vi "SyncParameters.vi"(4 "Excitation":T1={"Frequency"=1000.0, "Amplitude"=5e-07, "DC Offset"=0.0, "Cut Off"=40.0, "RaPF"=FALSE, "Shift"=0.0} {"Shift" min=-100.0 max=100.0 format="%_1p%"}, 6 "lineFitThreshold":dbl, 7 "inputSensitivity":dbl, 8 "error in":errorcluster, 9 "syncParameters":T4, 10 "BackgroundParameters":T3, 11 "FPGA VI Reference In":T2) -> (0 "error out":errorcluster, 3 "FPGA VI Reference Out":T2)   [LabVIEW 2016]
uses:
  controls/FPGAVIreferenceTypeDef.ctl
  controls/Enum.ctl
  <vilib>/Utility/error.llb/Error Cluster From Error Code.vi
  <vilib>/rvi/errors/niLvFpgaAdjustHostInterfaceError.vi
  <vilib>/rvi/interface/nirviReadWriteControl/nirviReadWriteControl.xnode
  FPGA Bitfiles/qnmController797_usbRIO_controllerFPGAmu.lvbitx
  NiFpgaLv.dll
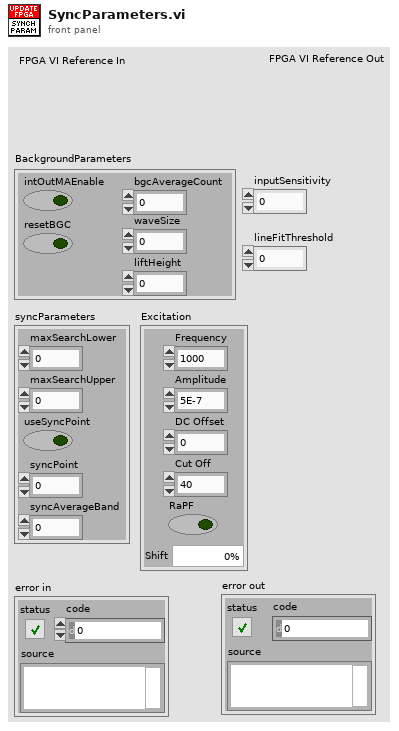
[diagram p1: front panel]
types:
  T1 = cluster{"Frequency":dbl, "Amplitude":dbl, "DC Offset":dbl, "Cut Off":dbl, "RaPF":bool, "Shift":dbl}
  T2 = typedef "FPGAVIreferenceTypeDef.ctl" = refnum<k20>
  T3 = cluster{"intOutMAEnable":bool, "bgcAverageCount":u16, "waveSize":u32, "resetBGC":bool, "liftHeight":fxp<+/-,15,4>}
  T4 = cluster{"maxSearchLower":u16, "maxSearchUpper":u16, "useSyncPoint":bool, "syncPoint":u16, "syncAverageBand":u16}
  T5 = typedef "Enum.ctl" = enum16{"Init", "Read", "Write"}
  T6 = cluster{"maxSearchLower":u16, "maxSearchUpper":u16}
  T7 = cluster{"ort.p.winSizeP2":u16, "ort.p.syncPoint":u16, "ort.p.useSyncPoint":bool, "ort.p.bypassAvg":bool, "ort.p.searchBounds":cluster{"maxSearchLower":u16, "maxSearchUpper":u16}}
  T8 = cluster{"maxLoc":u16, "threshold":i16, "fitHardPtLimit":u16}
  T9 = cluster{"liftHeight":fxp<+/-,15,4>, "disengagePos":fxp<+/-,22,1>}
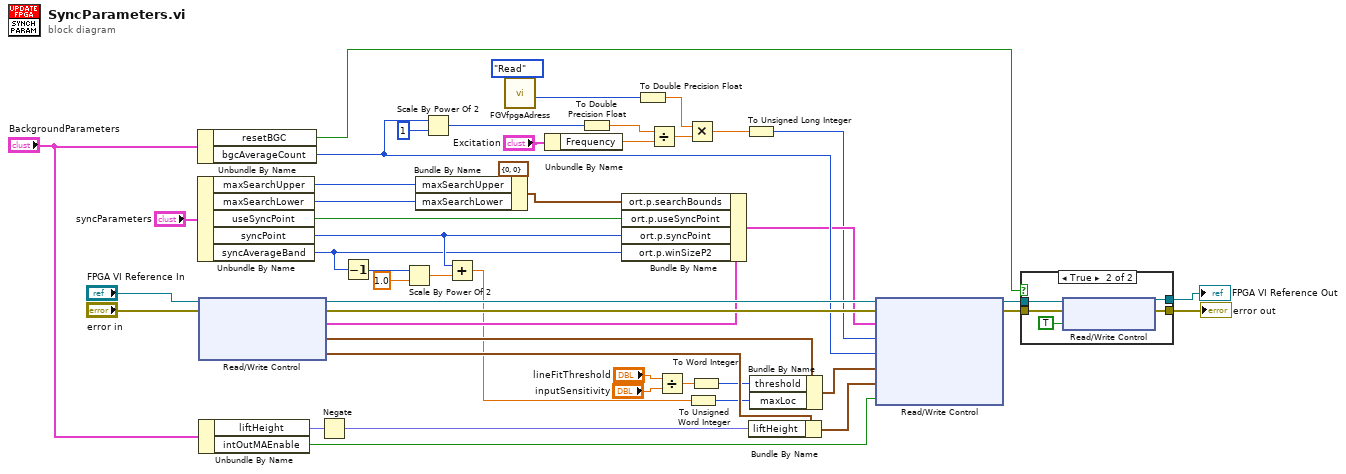
[diagram p0: block diagram]
diagram:
  n1 = Unbundle By Name("BackgroundParameters") -> ("resetBGC"=w40:bool, "bgcAverageCount"=w22:u16)
  n2 = Unbundle By Name("syncParameters") -> ("maxSearchUpper"=w46:u16, "maxSearchLower"=w47:u16, "useSyncPoint"=w24:bool, "syncPoint"=w16:u16, "syncAverageBand"=w14:u16)
  n3 = xnode ("Read/Write Control")("FPGA VI Reference In"="FPGA VI Reference In", "error in"="error in") -> ("FPGA VI Reference Out"=w29:T2, "error out"=w28:errorcluster, "ort.p.methodParams"=w27:T7, "ort.fit.p.params"=w26:T8, "fb.loff.p.params"=w19:T9)
  n4 = Unbundle By Name("BackgroundParameters") -> ("liftHeight"=w38:fxp<+/-,15,4>, "intOutMAEnable"=w8:bool)
  n5 = Negate(x=w38) -> (-x=w17:fxp<+/-,15,4>)
  n6 = Decrement(x=w14) -> (x-1=w43:u16)
  n7 = Scale By Power Of 2(n=w43, x=1.0) -> (x*2^n=w15:dbl)
  n8 = Bundle By Name(cluster=T6 {"maxSearchLower"=0, "maxSearchUpper"=0} ("maxSearchBounds"), "maxSearchUpper"=w46, "maxSearchLower"=w47) -> (w25:T6)
  n9 = Scale By Power Of 2(n=w22, x=u32 1) -> (x*2^n=w31:u32)
  n10 = Add(x=w16, y=w15) -> (x+y=w4:dbl)
  n11 = call "FGVfpgaAdress.vi"("Enum"=Enum."Read") -> ("baseClockOut"=w7:u32)  [unwired: 5 in, 5 out]
  n12 = Unbundle By Name("Excitation") -> ("Frequency"=w32:dbl)
  n13 = To Double Precision Float(number=w31) -> (double precision float=w2:dbl)
  n14 = Bundle By Name(cluster=w27, "ort.p.searchBounds"=w25, "ort.p.useSyncPoint"=w24, "ort.p.syncPoint"=w16, "ort.p.winSizeP2"=w14) -> (w12:T7)
  n15 = To Double Precision Float(number=w7) -> (double precision float=w1:dbl)
  n16 = Divide(x=w2, y=w32) -> (x/y=w13:dbl)
  n17 = Divide(x="lineFitThreshold", y="inputSensitivity") -> (x/y=w9:dbl)
  n18 = Multiply(x=w1, y=w13) -> (x*y=w23:dbl)
  n19 = To Unsigned Word Integer(number=w4) -> (unsigned 16bit integer=w3:u16)
  n20 = To Word Integer(number=w9) -> (16bit integer=w5:i16)
  n21 = To Unsigned Long Integer(number=w23) -> (unsigned 32bit integer=w6:u32)
  n22 = Bundle By Name(cluster=w19, "liftHeight"=w17) -> (w18:T9)
  n23 = Bundle By Name(cluster=w26, "threshold"=w5, "maxLoc"=w3) -> (w30:T8)
  n24 = xnode ("Read/Write Control")("FPGA VI Reference In"=w29, "error in"=w28, "ort.p.methodParams"=w12, "ort.bgc.p.waitTicks"=w6, "ort.bgc.p.bgCntP2"=w22, "ort.fit.p.params"=w30, "fb.loff.p.params"=w18, "ort.p.fcAvgEnable"=w8) -> ("FPGA VI Reference Out"=w11:T2, "error out"=w10:errorcluster)
  n25 = case shown="True" w40 {
    tunnel: w11 -> [w50 w54]
    tunnel: w10 -> [w49 w53]
    tunnel: [w50 w52] -> w35
    tunnel: [w49 w51] -> w37
    frame False {
    }
    frame True {
      n26 = xnode "Read/Write Control"("FPGA VI Reference In"=w54, "error in"=w53, "ort.bgc.p.start"=TRUE ("resetBGC")) -> ("FPGA VI Reference Out"=w52:T2, "error out"=w51:errorcluster)
    }
  }
  "error out" <- w37
  "FPGA VI Reference Out" <- w35
